vi "Initialize.vi"(8 "Error In":errorcluster, 11 "VI Path":path) -> (0 "Error Out":errorcluster, 2 "Message Queues":T2, 3 "Executable Configuration":T1)   [LabVIEW 2012]
uses:
  ActionQueues.ctl
  UIActionQueueElement.ctl
  UIAction.ctl
  HardwareActionQueueElement.ctl
  HardwareAction.ctl
  ExecutableConfiguration.ctl
  libs/LV-Utilities/LV-Utilities.lvlib
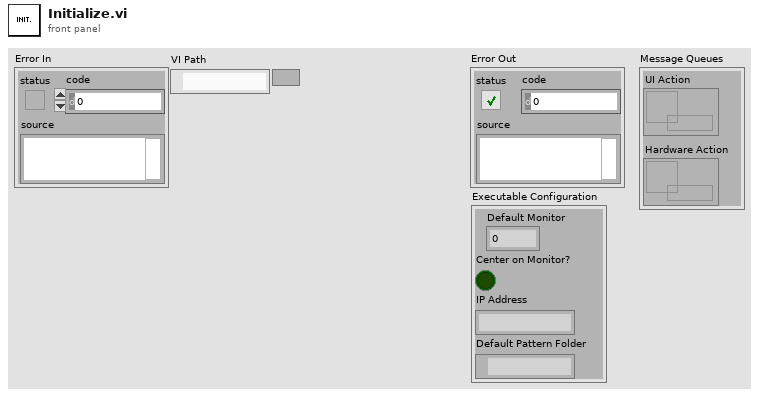
[diagram p1: front panel]
types:
  T1 = typedef "ExecutableConfiguration.ctl" = cluster{"Default Monitor":i32, "Center on Monitor?":bool, "IP Address":string, "Default Pattern Folder":path}
  T2 = typedef "ActionQueues.ctl" = cluster{"UI Action":refnum<queue>, "Hardware Action":refnum<queue>}
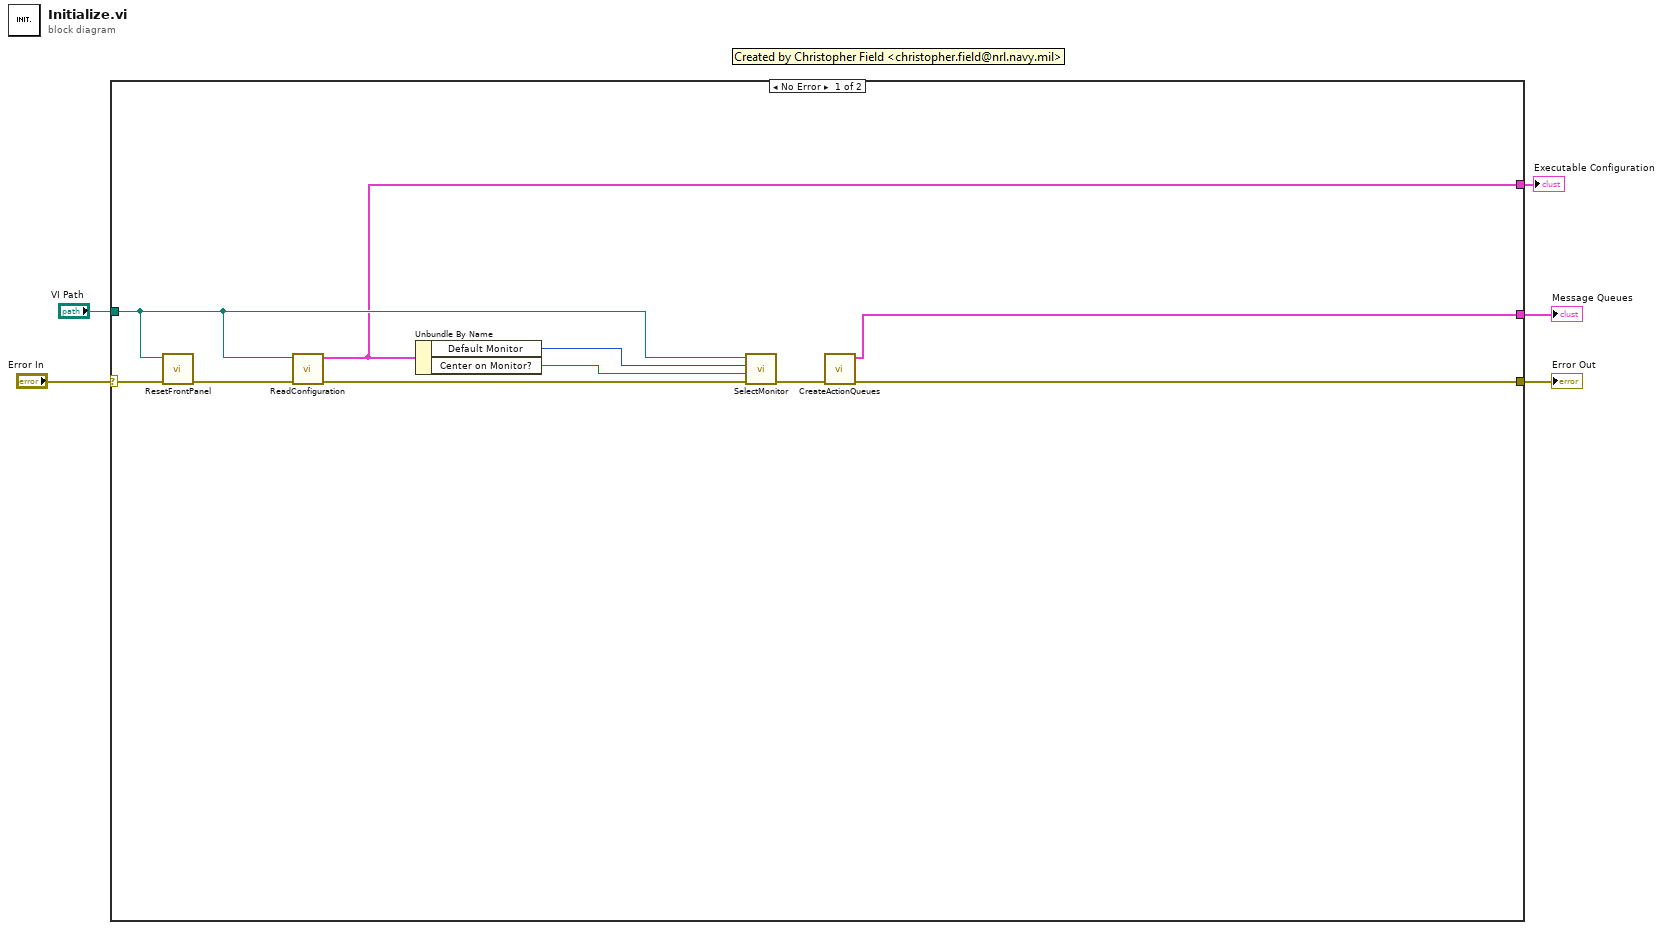
[diagram p0: block diagram]
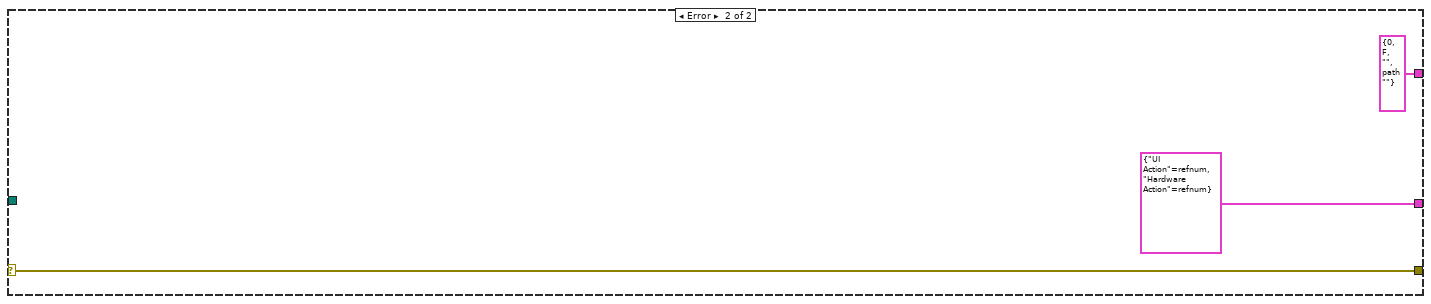
[diagram p2: hidden frame]
diagram:
  n1 = case shown="No Error" "Error In" {
    selector: "Error In" -> [w15 w18]
    tunnel: "VI Path" -> [w7 _]
    tunnel: [w14 w18] -> w3
    tunnel: [w13 T2 {"UI Action"=refnum, "Hardware Action"=refnum} ("Message Queues")] -> w2
    tunnel: [w6 T1 {"Default Monitor"=0, "Center on Monitor?"=FALSE, "IP Address"="", "Default Pattern Folder"=path ""} ("Executable Configuration")] -> w1
    frame No Error {
      n2 = call "ResetFrontPanel.vi"("Error In"=w15, "VI Path"=w7) -> ("Error Out"=w11:errorcluster)  [unwired: 9 in]
      n3 = call "ReadConfiguration.vi"("Error In"=w11, "VI Path"=w7) -> ("Error Out"=w10:errorcluster, "Executable Configuration"=w6:T1)  [unwired: 8 in]
      n4 = Unbundle By Name(w6) -> ("Default Monitor"=w9:i32, "Center on Monitor?"=w8:bool)
      n5 = call "SelectMonitor.vi"("Error In"=w10, "Center?"=w8, "Monitor (0=primary)"=w9, "VI Path"=w7) -> ("Error out"=w12:errorcluster)  [unwired: 7 in]
      n6 = call "CreateActionQueues.vi"("Error In"=w12) -> ("Error Out"=w14:errorcluster, "Message Queues"=w13:T2)  [unwired: 9 in]
    }
    frame Error {
    }
  }
  "Error Out" <- w3
  "Message Queues" <- w2
  "Executable Configuration" <- w1
